vi "Generate_Random_Params.vi"(7 "sampling info":cluster{"Fs":dbl, "#s":dbl}={"Fs"=10000.0, "#s"=2000.0}, 8 "Amplitude Range":cluster{"max":dbl, "min":dbl}={"max"=50.0, "min"=150.0}, 10 "Duration Range":cluster{"max":dbl, "min":dbl}={"max"=600.0, "min"=200.0}, 11 "Dataset Samples":i32=3000) -> (0 "Duration":i32[](array[numeric]), 1 "Amplitude":sgl[](array[numeric]), 2 "Position":dbl[](array[numeric]))   [LabVIEW 2020]
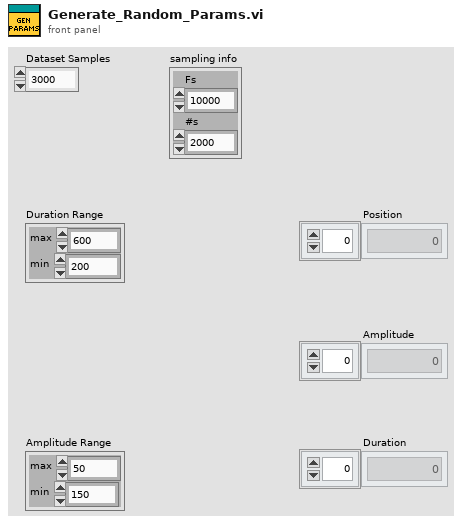
[diagram p1: front panel]
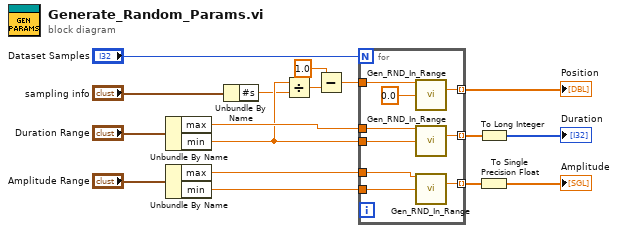
[diagram p0: block diagram]
diagram:
  n1 = Unbundle By Name("Duration Range") -> ("max"=w17:dbl, "min"=w16:dbl)
  n2 = Unbundle By Name("Amplitude Range") -> ("max"=w13:dbl, "min"=w14:dbl)
  n3 = Unbundle By Name("sampling info") -> ("#s"=w3:dbl)
  n4 = Divide(x=w16, y=w3) -> (x/y=w8:dbl)
  n5 = Subtract(x=1.0 ("end"), y=w8) -> (x-y=w1:dbl)
  n6 = for {
    N: "Dataset Samples" -> [_]
    tunnel: w14 -> [w26]
    tunnel: w13 -> [w25]
    tunnel: w17 -> [w24]
    tunnel: w16 -> [w23]
    tunnel: [w22] -> w9 mode=indexing
    tunnel: [w21] -> w10 mode=indexing
    tunnel: [w20] -> w2 mode=indexing
    tunnel: w1 -> [w18]
    n7 = call "Gen_RND_In_Range.vi"("Upper Bound"=w18, "Lower Bound"=0.0 ("end")) -> ("RND_In_Range"=w20:dbl)  [unwired: 13 in]
    n8 = call "Gen_RND_In_Range.vi"("Upper Bound"=w24, "Lower Bound"=w23) -> ("RND_In_Range"=w21:dbl)  [unwired: 13 in]
    n9 = call "Gen_RND_In_Range.vi"("Upper Bound"=w25, "Lower Bound"=w26) -> ("RND_In_Range"=w22:dbl)  [unwired: 13 in]
  }
  "Position" <- w2
  n10 = To Long Integer(number=w10) -> (32bit integer=→"Duration":i32[])
  n11 = To Single Precision Float(number=w9) -> (single precision float=→"Amplitude":sgl[])
